vi "Fuzzy_PT100_V4.vi"() -> ()   [LabVIEW 2025]
uses:
  <vilib>/DAQmx/write.llb/DAQmx Write (Digital 1D Bool 1Chan 1Samp).vi
  <vilib>/addons/Fuzzy Logic/FL Fuzzy Controller (SISO).vi
  <vilib>/DAQmx/create/channels.llb/DAQmx Create Channel (DO-Digital Output).vi
  <vilib>/DAQmx/miscellaneous.llb/DAQmx Fill In Error Info.vi
  <vilib>/Utility/file.llb/Write Delimited Spreadsheet (DBL).vi
  <vilib>/addons/Fuzzy Logic/NI_Fuzzy_Logic_API.lvlib
  <resource>/objmgr/daqmx.rc
panel:
  in  "Stop excel":bool
  out "Low Time":dbl
  out "High Time":dbl
  in  "Digital Lines":tag
  in  "stop 2":bool
  out "Waveform Chart":dynamicdata(graph)
  out "Duty":dbl
  out "Error":dbl
  in  "Temp Deseada":dbl
  out "Temp":dbl
  in  "file path":path
  out "data":dbl
  in  "Stop Fuzzy":bool
  # "Instituto Politécnico Nacional Unidad\n Profesional Interdisciplinaria \nDe Ingeniería \nCampus Zacatecas"
  # "Control con logica difusa"
  # "Integrantes :\nDiego Perez Dominguez\nDaniel Acevedo\nDaniel Alejandro Salas Serna"
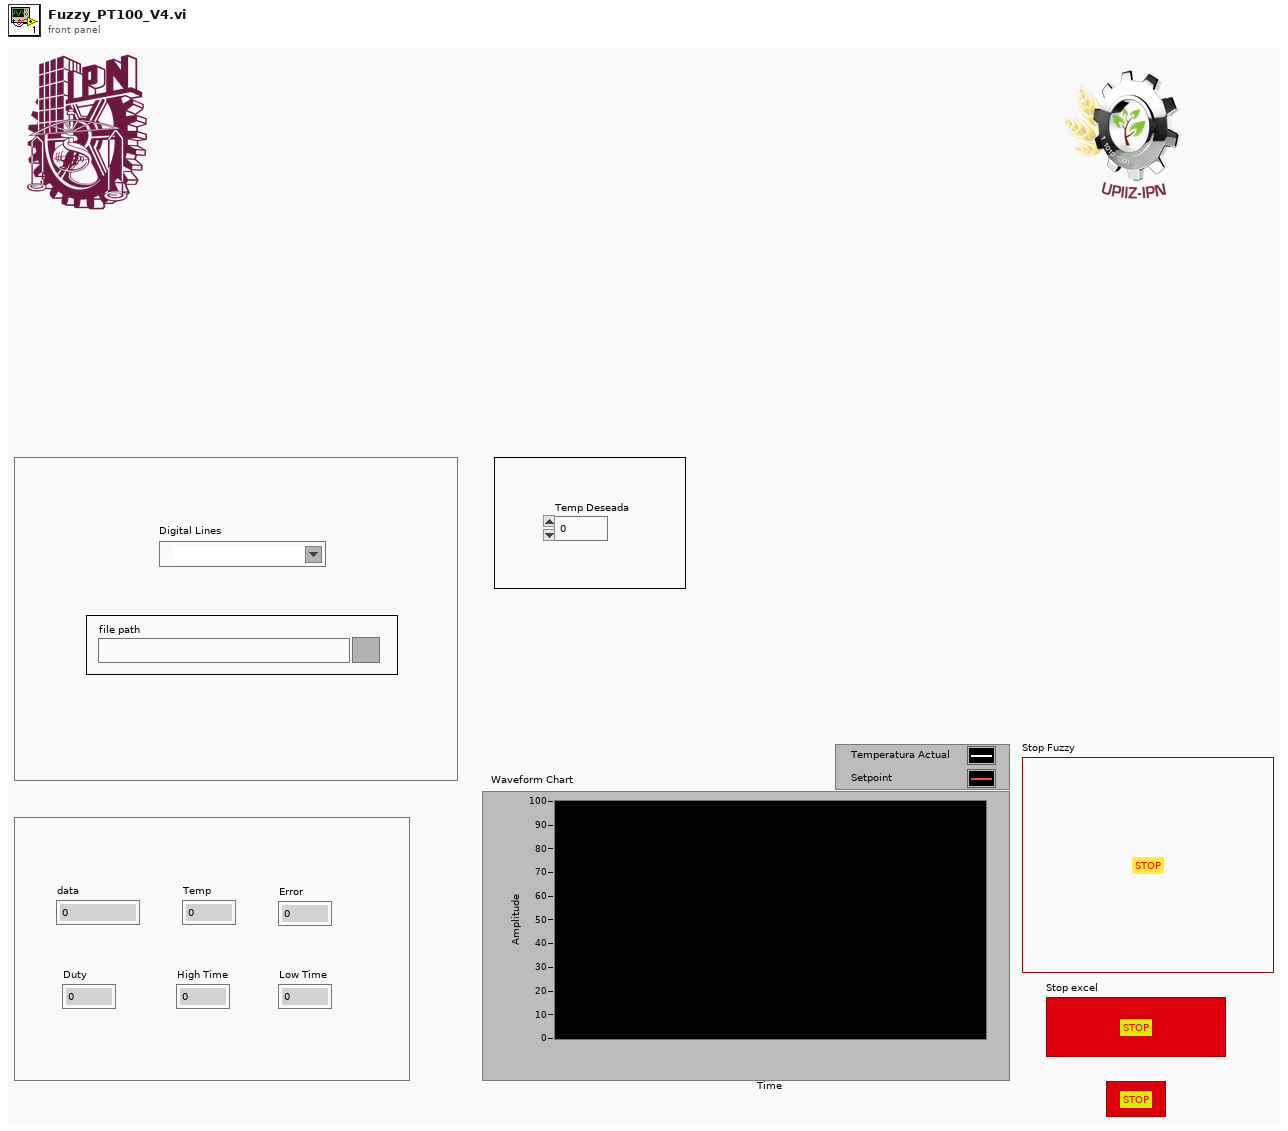
[diagram p1: front panel]
types:
  T1 = typedef "NI_Fuzzy_Logic_API.lvlib/FL System.ctl" = cluster{"input variables":T2[], "output variables":T2[], "rules":T5[], "defuzzification method":T11, "description":string, "user MF interpolating polynomials":T12[]}
  T2 = typedef "NI_Fuzzy_Logic_API.lvlib/FL Variable.ctl" = cluster{"name":string, "range":dbl[], "MFs":T3[]}
  T3 = typedef "NI_Fuzzy_Logic_API.lvlib/FL Membership Function.ctl" = cluster{"name":string, "shape":T4, "points":dbl[], "color":u32, "user-defined shape index":i32}
  T4 = typedef "NI_Fuzzy_Logic_API.lvlib/FL Membership Function Shape.ctl" = u16
  T5 = typedef "NI_Fuzzy_Logic_API.lvlib/FL Rule.ctl" = cluster{"antecedents":T6[], "antecedent connective":T8, "consequents":T9[], "consequent implication":T10, "degree of support":dbl}
  T6 = typedef "NI_Fuzzy_Logic_API.lvlib/FL Antecedent.ctl" = cluster{"Var Index":i32, "MF Index":i32, "Cond":T7}
  T7 = typedef "NI_Fuzzy_Logic_API.lvlib/FL Modifier.ctl" = u16
  T8 = typedef "NI_Fuzzy_Logic_API.lvlib/FL Antecedent Connective.ctl" = u16
  T9 = typedef "NI_Fuzzy_Logic_API.lvlib/FL Consequent.ctl" = cluster{"Var Index":i32, "MF Index":i32, "Cond":T7}
  T10 = typedef "NI_Fuzzy_Logic_API.lvlib/FL Consequent Implication.ctl" = u16
  T11 = typedef "NI_Fuzzy_Logic_API.lvlib/FL Defuzzification.ctl" = u16
  T12 = typedef "NI_Fuzzy_Logic_API.lvlib/FL Interpolating polynomials.ctl" = cluster{"X":dbl[], "Y":dbl[], "Y(x) coeff":dbl[][], "X(y) coeff":dbl[][], "Area(y) coeff":dbl[][], "coa_x(y) coeff":dbl[][]}
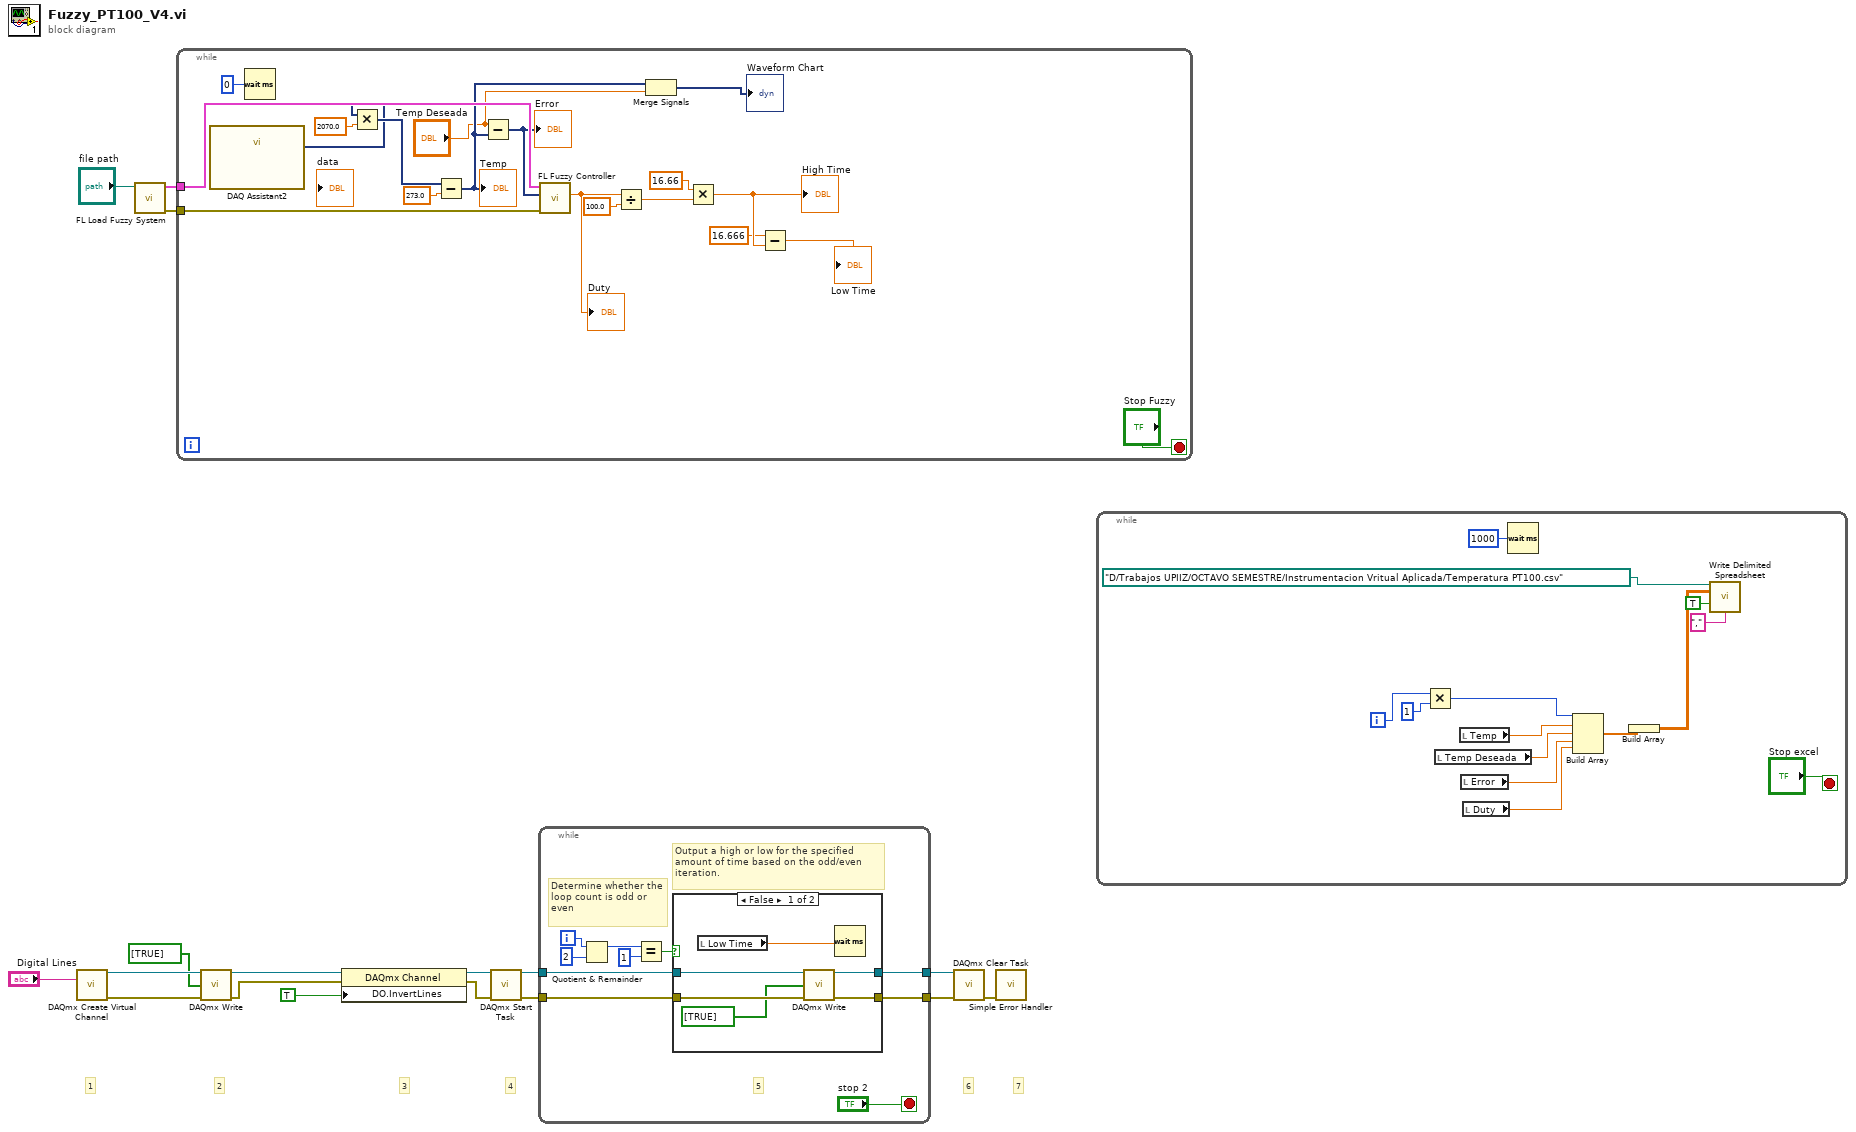
[diagram p0: block diagram]
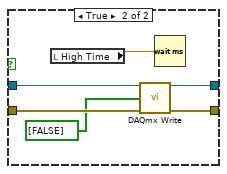
[diagram p2: hidden frame]
diagram:
  # "7"
  # "6"
  # "4"
  # "3"
  # "2"
  # "1"
  n1 = call-poly <vilib>:"DAQmx Create Virtual Channel.vi"("lines"="Digital Lines") -> ("task out"=w14:refnum<k21>, "error out"=w13:errorcluster)  [unwired: 13 in]
  n2 = call <vilib>:"FL Load Fuzzy System.vi"("file path"="file path") -> ("error out"=w15:errorcluster, "fuzzy system out"=w16:T1)  [unwired: 9 in]
  n3 = while {
    tunnel: w16 -> [w34]
    tunnel: w15 -> [w33]
    stop <- "Stop Fuzzy" stop-if-true
    n4 = call "DAQ Assistant2"() -> ("data"=w18:dynamicdata)  [unwired: 17 in, 2 out]
    n5 = Wait (ms)(milliseconds to wait=u32 0 ("millisecond timer value")) -> ()  [unwired: 1 out]
    n6 = Multiply(x=w18, y=2070.0) -> (x*y=w30:dynamicdata)
    n7 = Subtract(x=w30, y=273.0) -> (x-y=w24:dynamicdata)
    "Temp" <- w24
    n8 = Subtract(x="Temp Deseada", y=w24) -> (x-y=w25:dynamicdata)
    "Error" <- w25
    n9 = call-poly <vilib>:"FL Fuzzy Controller.vi"("error in (no error)"=w33, "input value"=w25, "fuzzy system in"=w34) -> ("output value"=w22:dbl)  [unwired: 4 in, 4 out]
    "Duty" <- w22
    n10 = Divide(x=w22, y=100.0) -> (x/y=w27:dbl)
    n11 = Merge Signals(w24, "Temp Deseada") -> (→"Waveform Chart":dynamicdata)
    n12 = Multiply(x=16.66 ("y"), y=w27) -> (x*y=w21:dbl)
    "High Time" <- w21
    n13 = Subtract(x=16.666, y=w21) -> (x-y=→"Low Time":dbl)
  }
  n14 = call-poly <vilib>:"DAQmx Write.vi"("task/channels in"=w14, "data"=bool[] [TRUE], "error in"=w13) -> ("task out"=w5:refnum<k21>, "error out"=w1:errorcluster)  [unwired: 10 in, 1 out]
  n15 = property class="DAQmx Channel"(reference=w5, error in=w1, "DO.InvertLines"=TRUE) -> (reference out=w4:refnum<k21>, error out=w3:errorcluster)
  n16 = call <vilib>:"DAQmx Start Task.vi"("task/channels in"=w4, "error in"=w3) -> ("task out"=w12:refnum<k21>, "error out"=w11:errorcluster)  [unwired: 12 in]
  n17 = while {
    tunnel: w12 -> [w46]
    tunnel: w11 -> [w45]
    tunnel: [w44] -> w10
    tunnel: [w43] -> w9
    i -> [w41]
    stop <- "stop 2" stop-if-true
    # "5"
    # "Output a high or low for the specified\namount of time based on the odd/even\niteration."
    # "Determine whether the loop count is odd or even"
    n18 = Quotient & Remainder(x=w41, y=2) -> (x-y*floor(x/y)=w39:i32)  [unwired: 1 out]
    n19 = Equal?(x=w39, y=1) -> (x = y?=w37:bool)
    n20 = case shown="False" w37 {
      tunnel: w46 -> [w50 w58]
      tunnel: w45 -> [w49 w57]
      tunnel: [w51 w56] -> w44
      tunnel: [w52 w55] -> w43
      frame False {
        n21 = local read "Low Time"() -> (w47:dbl)
        n22 = call-poly <vilib>:"DAQmx Write.vi"("task/channels in"=w50, "data"=bool[] [TRUE], "error in"=w49) -> ("task out"=w52:refnum<k21>, "error out"=w51:errorcluster)  [unwired: 10 in, 1 out]
        n23 = Wait (ms)(milliseconds to wait=w47) -> ()  [unwired: 1 out]
      }
      frame True {
        n24 = local read "High Time"() -> (w53:dbl)
        n25 = call-poly <vilib>:"DAQmx Write.vi"("task/channels in"=w58, "data"=bool[] [FALSE], "error in"=w57) -> ("task out"=w55:refnum<k21>, "error out"=w56:errorcluster)  [unwired: 10 in, 1 out]
        n26 = Wait (ms)(milliseconds to wait=w53) -> ()  [unwired: 1 out]
      }
    }
  }
  n27 = call <vilib>:"DAQmx Clear Task.vi"("task in"=w9, "error in"=w10) -> ("error out"=w8:errorcluster)  [unwired: 13 in]
  n28 = call <vilib>:"Simple Error Handler.vi"("error in (no error)"=w8) -> ()  [unwired: 4 in, 5 out]
  n29 = while {
    i -> [w70]
    stop <- "Stop excel" stop-if-true
    n30 = Multiply(x=w70, y=1) -> (x*y=w63:i32)
    n31 = local read "Temp Deseada"() -> (w61:dbl)
    n32 = local read "Temp"() -> (w62:dbl)
    n33 = local read "Error"() -> (w60:dbl)
    n34 = local read "Duty"() -> (w59:dbl)
    n35 = Wait (ms)(milliseconds to wait=u32 1000) -> ()  [unwired: 1 out]
    n36 = Build Array(w63, w62, w61, w60, w59) -> (w68:dbl[])
    n37 = Build Array(w68) -> (w67:dbl[][])
    n38 = call-poly <vilib>:"Write Delimited Spreadsheet.vi"("file path (dialog if empty)"=path "D:/Trabajos UPIIZ/OCTAVO SEMESTRE/Instrumentacion Vritual Aplicada/Temperatura PT100.csv" ("name or relative path"), "2D data"=w67, "append to file? (new file:F)"=TRUE, "delimiter (\\t)"="," ("delimiter (\\t)")) -> ()  [unwired: 10 in, 2 out]
  }
